vi "WPI_UtilitiesERRGetRefNum.vi"(8 "error in (no error)":errorcluster, 10 "unfound refnum name":string) -> (0 "ERRGetRefNum":errorcluster)   [LabVIEW 2025]
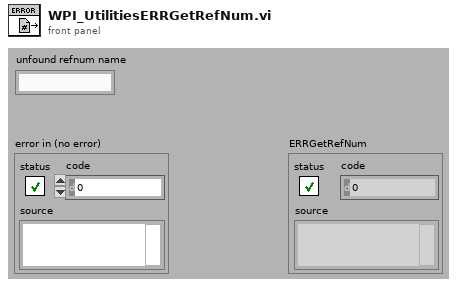
[diagram p1: front panel]
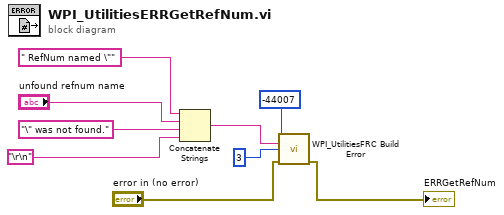
[diagram p0: block diagram]
diagram:
  n1 = Concatenate Strings(" RefNum named \"" ("unfound refnum name"), "unfound refnum name", "\" was not found." ("unfound refnum name"), "\r\n") -> (w5:string)
  n2 = call <vilib>:"WPI_UtilitiesFRC Build Error.vi"("error code"=-44007 ("code"), "extra error text"=w5, "chain levels to remove (1)"=3, "error in (no error)"="error in (no error)") -> ("error out"=→"ERRGetRefNum":errorcluster)  [unwired: 1 in, 10 out]
